vi "analog read.vi"(8 "error in (no error)":errorcluster, 10 "Line":string, 11 "USB-6000 in":refnum<class "USB-6000.lvclass">) -> (0 "error out":errorcluster, 2 "Voltage":dbl, 3 "USB-6000 out":refnum<class "USB-6000.lvclass">)   [LabVIEW 2025, in "USB IO.lvlib" / "USB-6000.lvclass"]
uses:
  USB-6000.lvclass
  USB-6000.lvclass/USB-6000.ctl
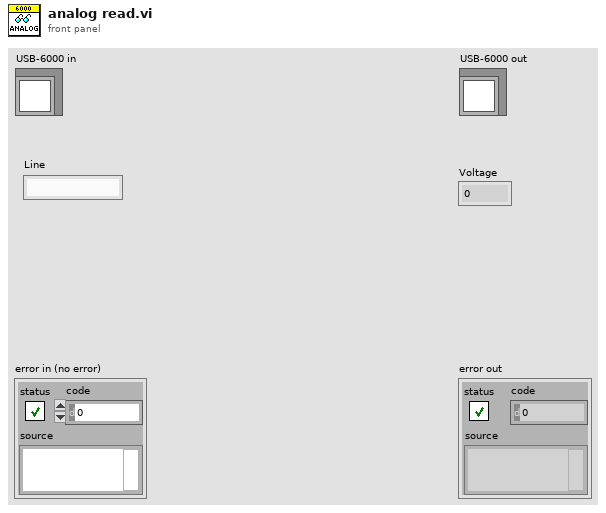
[diagram p1: front panel]
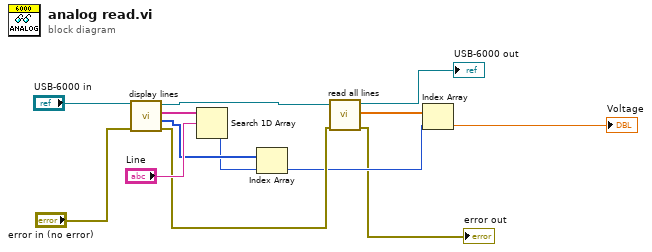
[diagram p0: block diagram]
diagram:
  n1 = call-dynamic "display lines.vi"("error in (no error)"="error in (no error)", "USB-6000 in"="USB-6000 in") -> ("error out"=w6:errorcluster, "Values"=w9:i32[], "Lines"=w11:string[], "USB-6000 out"=w7:refnum<class "USB-6000.lvclass">)  [unwired: 6 in]
  n2 = Search 1D Array(1D array=w11, element="Line") -> (index of element=w8:i32)  [unwired: 1 in]
  n3 = Index Array(array=w9, index=w8) -> (element=w4:i32)
  n4 = call-dynamic "read all lines.vi"("error in (no error)"=w6, "USB-6000 in"=w7) -> ("error out"=→"error out":errorcluster, "Array"=w5:dbl[], "USB-6000 out"=→"USB-6000 out":refnum<class "USB-6000.lvclass">)  [unwired: 7 in]
  n5 = Index Array(array=w5, index=w4) -> (element=→"Voltage":dbl)
